vi "Download Bitfile Dynamic.vi"(0 "Target Info":cluster{"FPGA Target Resource":string}={"FPGA Target Resource"="rio://192.168.1.1/RIO0"}, 5 "Operation (0:Erase Flash)":enum16{"Erase Flash", "Download Bitfile"}(ring), 7 "Bitfile Path":path, 11 "Error In":errorcluster) -> (4 "Target Info Out":cluster{"FPGA Target Resource":string}, 15 "Error Out":errorcluster)   [LabVIEW 2020]
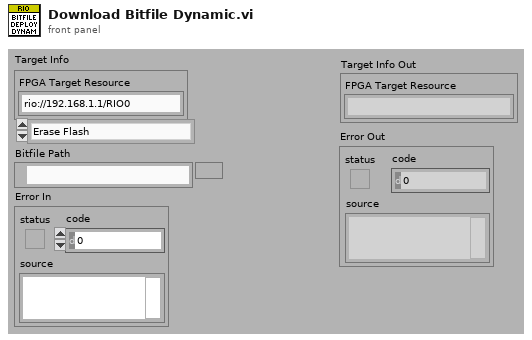
[diagram p1: front panel]
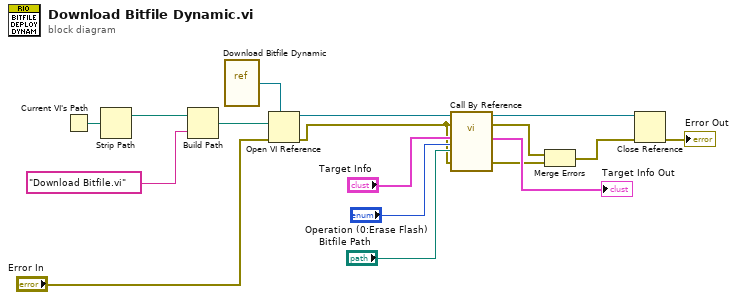
[diagram p0: block diagram]
diagram:
  n1 = Current VI's Path() -> (path=w1:path)
  n2 = Strip Path(path=w1) -> (stripped path=w14:path)  [unwired: 1 out]
  n3 = Build Path(base path=w14, name or relative path="Download Bitfile.vi") -> (appended path=w15:path)
  n4 = vi-ref "Download Bitfile Dynamic.vi"() -> (w16:refnum<vi>)
  n5 = Open VI Reference(type specifier VI Refnum (for type only)=w16, vi path=w15, error in (no error)="Error In") -> (vi reference=w17:refnum<vi>, error out=w6:errorcluster)  [unwired: 3 in]
  n6 = call-by-ref "?"(reference=w17, error in=w6, "Target Info"="Target Info", "Operation (0:Erase Flash)"="Operation (0:Erase Flash)", "Bitfile Path"="Bitfile Path", "Error In"=w6) -> (reference out=w7:refnum<vi>, error out=w5:errorcluster, "Target Info Out"=→"Target Info Out":cluster{"FPGA Target Resource":string}, "Error Out"=w4:errorcluster)  [unwired: 10 in]
  n7 = Merge Errors(w5, w4) -> (w3:errorcluster)
  n8 = Close Reference(reference=w7, error in (no error)=w3) -> (error out=→"Error Out":errorcluster)
